vi "Get DDG Gate Time.vi"(10 "puiWidth":cluster{}, 11 "puiDelay":cluster{}) -> (1 "function return":u32, 2 "puiWidth out":cluster{}, 3 "puiDelay out":cluster{})   [LabVIEW 2018, in "Copy of Andor SDK.lvlib"]
doc: "EXPNETTYPE unsigned int WINAPI GetDDGGateTime(at_u64 * puiDelay, at_u64 * puiWidth);"
uses:
  Copy of Andor SDK.lvlib
  <userlib>/Andor SDK/ATMCD32D.dll
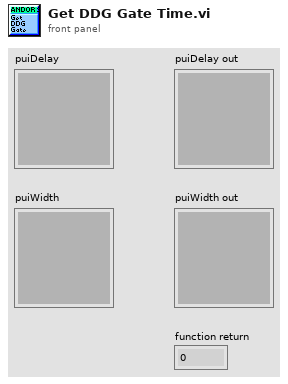
[diagram p1: front panel]
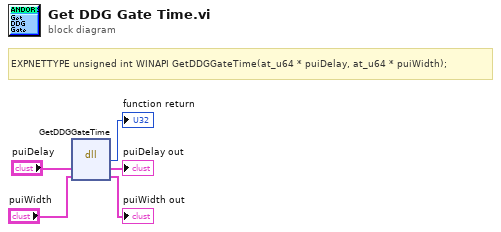
[diagram p0: block diagram]
diagram:
  # "EXPNETTYPE unsigned int WINAPI GetDDGGateTime(at_u64 * puiDelay, at_u64 * puiWidth);"
  n1 = dll-call lib="C:/Program Files (x86)/National Instruments/LabVIEW 2018/user.lib/Andor SDK/ATMCD32D.*" fn="GetDDGGateTime"("puiDelay"="puiDelay", "puiWidth"="puiWidth") -> (→"function return":u32, "puiDelay"=→"puiDelay out":cluster{}, "puiWidth"=→"puiWidth out":cluster{})  [unwired: 3 in, 2 out]
